vi "Read Current Position.vi"(4 "Units (0: microsteps)":u16(ring) items=["microsteps", "microns", "millimeters", "inches", "degrees"], 8 "error in (no error)":errorcluster, 9 "Device and Axis":string, 10 "Microstep Size (0)":dbl, 11 "VISA resource name":refnum<visa-resource-name>) -> (0 "error out":errorcluster, 2 "Position":dbl, 3 "VISA resource name out":refnum<visa-resource-name>)   [LabVIEW 2018, in "Zaber A Series.lvlib"]
doc: "Returns the current position. The unit of the value returned depends on the Units input (default is microsteps). For units other than microsteps, a Microstep Size is required for accurate results. You can optionally read from the position of a single device or axis by specifying the Device and Axis input.\n\nThis VI requires that the Initialize VI has been called with the same serial port."
uses:
  Zaber A Series.lvlib
  Utility/Low Level/Convert Device Units to Position Units (FW7).vi
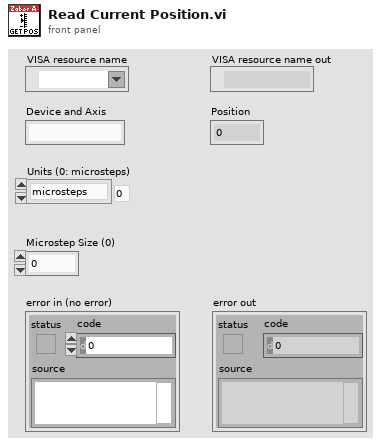
[diagram p1: front panel]
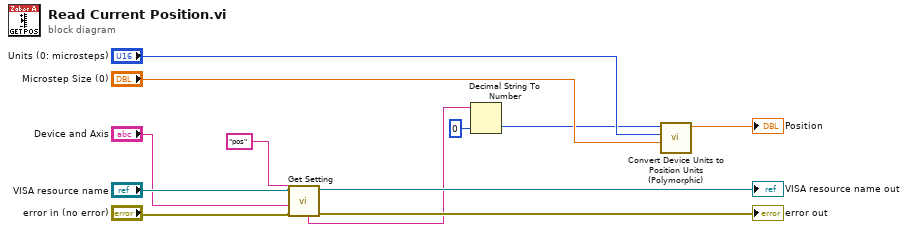
[diagram p0: block diagram]
diagram:
  n1 = call "Get Setting.vi"("error in (no error)"="error in (no error)", "Device and Axis"="Device and Axis", "Setting"="pos" ("All Settings (Access Level 2)"), "VISA resource name"="VISA resource name") -> ("error out"=→"error out":errorcluster, "VISA resource name out"=→"VISA resource name out":refnum<visa-resource-name>, "First Response Data"=w1:string)  [unwired: 2 in, 3 out]
  n2 = Decimal String To Number(string=w1, default (0L)=i64 0 ("default (0 I32)")) -> (number=w4:i64)  [unwired: 1 in, 1 out]
  n3 = call-poly "Convert Device Units to Position Units (Polymorphic).vi"("Microstep Size (0)"="Microstep Size (0)", "Units (0: microsteps)"="Units (0: microsteps)", "Device Position (0)"=w4) -> ("Position"=→"Position":dbl)  [unwired: 8 in]
